vi "Apply Device Order to Hardware Array.vi"(8 "error in (no error)":errorcluster, 10 "Compatible Hardware Types":string[](array[string]), 11 "Array of Hardware in":refnum<class "Hardware.lvclass">[](array[class])) -> (0 "error out":errorcluster, 3 "Array":refnum<class "Hardware.lvclass">[](array[class]))   [LabVIEW 2016, in "Hardware.lvlib" / "Hardware.lvclass"]
uses:
  <userlib>/Common Components/Hardware/Abstract Hardware/Hardware.lvclass
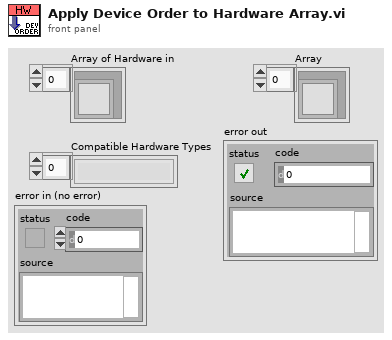
[diagram p1: front panel]
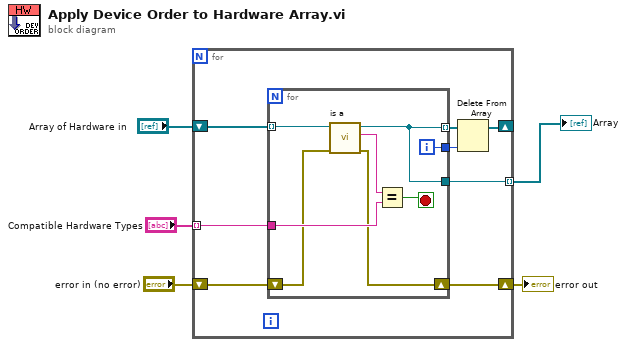
[diagram p0: block diagram]
diagram:
  n1 = for {
    tunnel: "Compatible Hardware Types" -> [w12] mode=indexing
    shift-right: [w8] -> _
    shift-left: "Array of Hardware in" -> [w13]
    tunnel: [w11] -> w4 mode=indexing
    shift-right: [w6] -> w1
    shift-left: "error in (no error)" -> [w7]
    n2 = for {
      tunnel: w13 -> [w21] mode=indexing
      tunnel: w12 -> [w20]
      tunnel: [w17] -> w11
      tunnel: [w17] -> w10 mode=indexing
      tunnel: [w16] -> w9
      shift-right: [w14] -> w6
      shift-left: w7 -> [w15]
      i -> [w16]
      stop <- w18 stop-if-true
      n3 = call-dynamic "is a.vi"("error in (no error)"=w15, "Hardware in"=w21) -> ("error out"=w14:errorcluster, "is a"=w19:string, "Hardware out"=w17:refnum<class "Hardware.lvclass">)  [unwired: 7 in]
      n4 = Equal?(x=w19, y=w20) -> (x = y?=w18:bool)
    }
    n5 = Delete From Array(array=w10, index=w9) -> (array with subset deleted=w8:refnum<class "Hardware.lvclass">[])  [unwired: 1 in, 1 out]
  }
  "Array" <- w4
  "error out" <- w1
